vi "File Popup For Save as.vi"(8 "error in (no error)":errorcluster) -> (0 "error out":errorcluster, 1 "exists":bool, 2 "cancelled":bool, 3 "selected path":path)   [LabVIEW 2021]
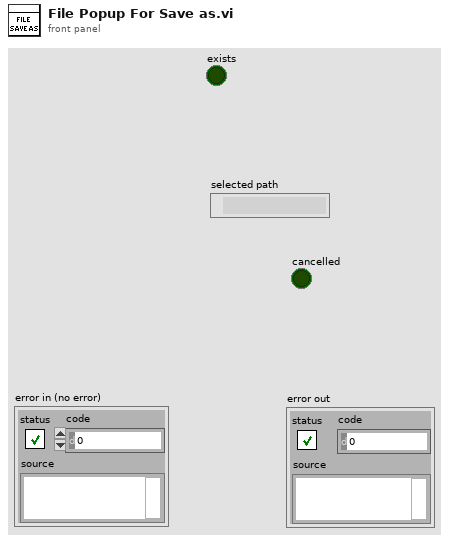
[diagram p1: front panel]
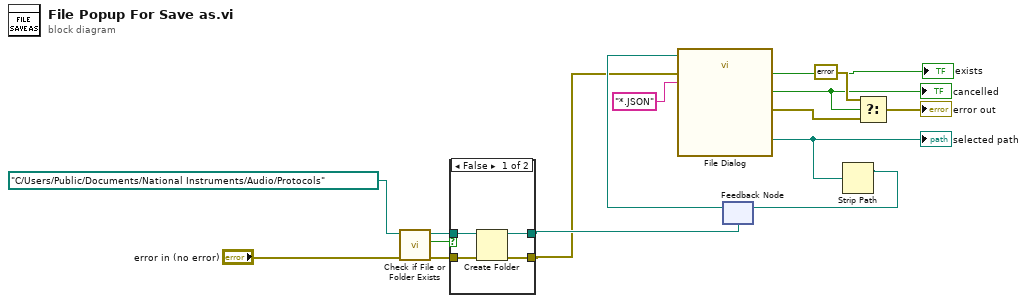
[diagram p0: block diagram]
diagram:
  n1 = call <vilib>:"Check if File or Folder Exists.vi"("error in (no error)"="error in (no error)", "path"=path "C:/Users/Public/Documents/National Instruments/Audio/Protocols") -> ("error out"=w15:errorcluster, "file or folder exists?"=w16:bool, "dup path"=w14:path)  [unwired: 7 in]
  n2 = case shown="False" w16 {
    tunnel: w15 -> [w20 w21]
    tunnel: w14 -> [w19 w22]
    tunnel: [w18 w22] -> w11
    tunnel: [w17 w21] -> w6
    frame False {
      n3 = Create Folder(path (use dialog)=w19, error in=w20) -> (created path=w18:path, error out=w17:errorcluster)  [unwired: 1 in, 1 out]
    }
    frame True {
    }
  }
  n4 = feedback #1(w11) -> (w7:path)
  n5 = call "File Dialog"("start path"=w7, "error in"=w6, "pattern (all files)"="*.JSON") -> ("selected path"=w2:path, "exists"=→"exists":bool, "cancelled"=w4:bool, "error out"=w3:errorcluster)  [unwired: 9 in]
  "cancelled" <- w4
  "selected path" <- w2
  n6 = Strip Path(path=w2) -> (stripped path=w12:path)  [unwired: 1 out]
  n7 = feedback-in #1(w12) -> ()
  n8 = Select(t=errorcluster {"status"=FALSE, "code"=0, "source"=""}, s=w4, f=w3) -> (s? t:f=→"error out":errorcluster)
